vi "knrm-robotics-ultrasonic-scan.vi"() -> ()   [LabVIEW 2015]
uses:
  <userlib>/KNR OS 3.0 LabVIEW Toolkit/Type Definition/Ultrasonic Port Number.ctl
  <userlib>/KNR OS 3.0 LabVIEW Toolkit/Type Definition/Resource.ctl
  <userlib>/KNR OS 3.0 LabVIEW Toolkit/Type Definition/RC Servo Port.ctl
  <vilib>/ptbypt/NI_PtbyPt.lvlib
panel:
  out "output array":u16[](array[numeric])
  in  "?":bool
  in  "?":bool
  out "x-y":u32
  in  "Port Number":T1 items=["US1-US4"=0, "US5-US8"=2]
  in  "RC Pulse Width (uS)":u16[](array[numeric])=[1500, 1500, 1500, 1500, 1500, 1500, 1500]
  out "US":dbl(slide)=299.99420158565044 scale=0.0..300.0
  out "Ultrasonic output":T2
  out "XY Graph":cluster{dbl[], dbl[]}(graph)={[52.83510722219944, 52.41501941107636, 18.825090961382138, 18.810750829633513, 18.842068219739453, 18.867520707739345, 18.86999233966576, 19.343794430132927, 19.299396729094312, 19.249120244854563, 19.192980292117813, 19.56923700536949, 19.550257015140925, 20.0268746752987, 19.94313209159437, 19.853314636661487, 19.757449669766896, 20.476600911619304, 32.61215421079407, 32.42225574220841, 32.62586723383785, 32.42968403430184, 32.65326536183423, 33.19253900698759, 32.94158974146576, 33.80108407369108, 37.79584583915372, 37.468367050903275, 36.76560921195627, 36.403821071494754, 35.70408342661834, 35.309448959916324, 30.390512880027405, 33.7842674842371, 33.026100281524855, 32.632293705492096, 31.8534734091588, 31.444722619895053, 31.310542727675877, 30.878844889448313, 29.345981113135775, 28.61370061639986, 28.17523999703333, 27.351455120555766, 26.58100847356183, 26.092549408742254, 25.633197609818932, 25.16603769058929, 25.173776355470487, 24.6820024593776, 24.149598305560747, 23.64363348068164, 22.855607283966688, 22.072898695449073, 21.548232931052418, 20.99779051069682, 20.4712305073856, 19.938434768952572, 19.39956559014096, 18.837099698165826, 18.287094309926037, 17.731518495608384, 17.1463576277358, 16.58094778294143, 16.010487220829134, 15.253730460161847, 14.68050882655889, 14.08939689452119, 13.50152896715735, 12.916257579894289, 12.327051775449814, 11.734091031619695, 11.13755596999065, 10.537628300921224, 9.934490768191035, 9.328327093335284, 8.731784028189727, 8.119248646656601, 7.504240063332757, 6.8869456157904345, 6.2675533378981925, 5.6543103020243946, 5.030399780002455, 4.3631046269165985, 3.7422752021515957, 3.120305844107791, 2.496188223621293, 1.785636799859872, 1.1907267982129588, 0.5954540896484806, 2.066038963463892e-15, -0.5888612411470842, -1.163760162118542, -1.7451971139043094, -2.3249046746875894, -2.9018096075419657, -3.446123927161177, -4.017822965793698, -4.588298136629306, -5.157375667404677, -5.730845630561522, -6.375830717568115, -6.979443065564002, -7.555304639800326, -8.125294747449619, -8.692809811607347, -9.252943998005462, -9.814703824821812, -10.511433242759157, -97.66855855808836, -12.115630210935187, -14.780776897049115, -15.03243125118948, -16.11558635268566, -20.83347185044012, -21.98075621495253, -25.193747403909317, -26.09141148542781, -26.981127870254667, -27.86262554216021, -25.72212889790534, -26.495751500330893, -27.261303240179316, -28.018550922974622, -28.76726388373698, -29.260992311107042, -29.703255042663816, -30.153894378895316, -30.572810483455903, -31.251091419621243, -31.93089026416236, -32.61268695568148, -33.2624749197111, -33.90213081165937, -34.245188616933525, -34.85886894020428, -35.869539315624316, -36.46860682740769, -37.056565648272105, -37.633236680265036, -38.1984442638038, -38.75201623118319, -39.293783959019336, -39.823582419614134, -40.688540608559144, -41.198270803183775, -41.69545160542513, -42.698360226241675, -43.175788543019294, -43.64006509635344, -44.09104846310844, -44.874017063377195, -45.3012949795156, -45.760672049510696, -46.57732247552712, -46.966699693554176, -52.016338848904994, -52.90258478875593, -53.2864354783321, -57.421220074576965, -82.14554405908432, -82.65483424315623, -53.743915627302584, -54.04049206105783, -54.320607237429286, -54.252457958663086, -54.49789897377209, -55.06135718998163, -86.91802410081984, -87.22721920998029, -57.39292961361045, -57.56080538417302, -84.61127588015269, -87.43054222606335, -87.60457982125371, -65.41196662411174, -65.50188079298516, -67.25229239181644, -67.4580059883256, -67.33432889952226, -67.49912463128567], [0.0, 0.9149075670341228, 0.6573866621236092, 0.9858296776277172, 1.317565761028515, 1.6506941707678109, 1.9833161143297424, 2.375119305299923, 2.712353325559518, 3.048761136720991, 3.384240265706206, 3.8038743386930016, 4.155535410903584, 4.623568330184559, 4.972381294834969, 5.319679623974433, 5.665357527167541, 6.260325150666395, 10.596331239671903, 11.163877937181766, 11.874844540237977, 12.448589368330708, 13.192775565335738, 14.08939689452119, 14.666540692565961, 15.761704357503108, 18.434265728166686, 19.091086563433738, 19.548621178777296, 20.178967527396583, 20.613762177526947, 21.21605735957737, 18.990100087534795, 21.939759834879325, 22.276385917980576, 22.849378041658824, 23.142903096441774, 23.69529808458086, 24.462476991257596, 25.00519555498049, 24.62420192856765, 24.873510465680386, 25.36910004239107, 25.50564452773545, 25.668981505970372, 26.09254940874225, 26.543953164351468, 26.98727137468978, 27.958311065896748, 28.39339585621924, 28.780370540359066, 29.19745575545069, 29.25384329180434, 29.291725911947594, 29.65859822440211, 29.987952663840147, 30.349847327677153, 30.702497134012567, 31.0457946622992, 31.350198534648506, 31.674176467595604, 31.988506139556034, 32.24760857477566, 32.541942310033185, 32.8263634544222, 32.711730535404534, 32.972962684076684, 33.19253900698759, 33.41745684763044, 33.64800137815105, 33.86829640149636, 34.07827481366822, 34.277872653208185, 34.46702912068076, 34.64568659719358, 34.81379066194859, 35.02127289601618, 35.16832963030732, 35.30467375070981, 35.43026372548378, 35.545061298706294, 35.69991023384921, 35.79315428611765, 35.53463558310762, 35.60537016126978, 35.66525899876386, 35.69715469994275, 34.07197985276371, 34.09795418438132, 34.113541948840066, 33.74097682535648, 33.735837911157894, 33.32573076299372, 33.300344677436904, 33.247685831376614, 33.16783558686001, 32.787678997428294, 32.72254211969623, 32.64743763864413, 32.56238843182445, 32.50124063563915, 32.80080552321191, 32.835697993643045, 32.72561977016228, 32.5887772524299, 32.44200787745185, 32.26885054669531, 32.10244970506474, 32.350865043356556, 283.65009017131854, 33.28742042700667, 38.50524026218143, 37.20657296470336, 37.965942235611514, 46.79274390418685, 47.137883820999214, 51.65483708601368, 51.20727828475838, 50.744121250481506, 50.26550706530237, 44.55203413000772, 44.096335591458654, 43.62720488191764, 43.14478490314336, 42.649222604934685, 41.7890278444039, 40.8830232198667, 40.01556938720181, 39.13141295092422, 38.59188393270723, 38.05375318704697, 37.51660474840471, 36.94172092002333, 36.35558428558721, 35.46193091431041, 34.85886894020429, 34.638811474599436, 34.0075260369806, 33.365881577492594, 32.714073547253555, 32.05230049330367, 31.3807639981259, 30.699668618242033, 30.009221821902685, 29.561955154591352, 28.84733977759426, 28.123937221450483, 27.728639348003938, 26.979227005050628, 26.22159652819797, 25.45597869902849, 24.87407383327599, 24.087125807087233, 23.316226995194086, 22.717278059455737, 21.900931745370343, 23.159166160261293, 22.455814955220205, 21.52911741451913, 22.041941234483758, 29.89853291510958, 28.460341801798872, 17.46245673999011, 16.521836464188556, 15.576183476949357, 14.536902297427226, 13.587852310280022, 12.71191593536959, 18.474996350022376, 16.95525383525952, 10.119921992781398, 9.116735945401807, 11.891339337430969, 10.735120736730053, 9.207612367883806, 5.722805538545885, 4.580337700157324, 3.5245432959488956, 2.3556854774912677, 1.175325082839114, 8.266258692495226e-15]}
  in  "RC Power":bool
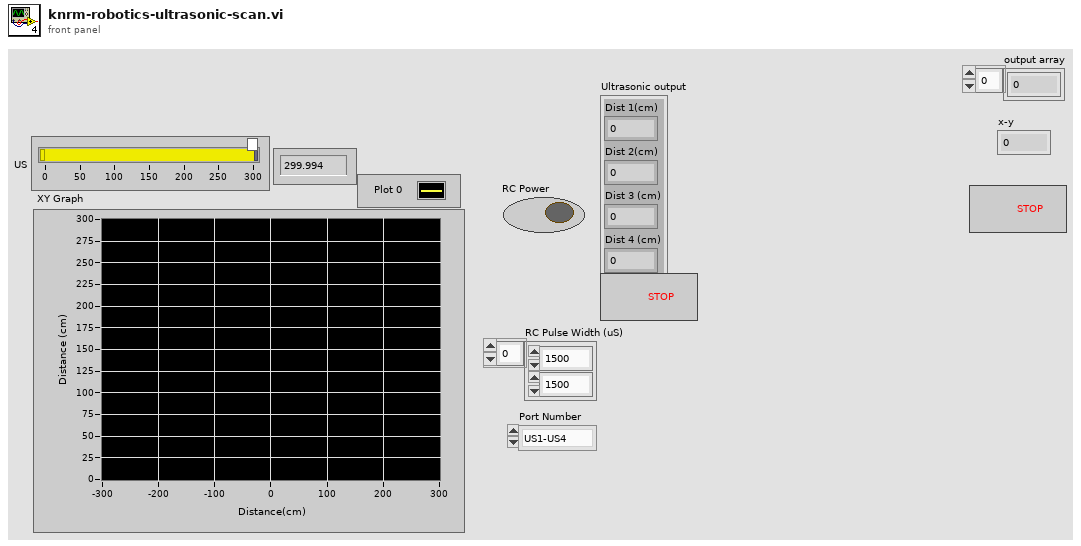
[diagram p1: front panel]
types:
  T1 = typedef "Ultrasonic Port Number.ctl" = u16
  T2 = cluster{"Dist 1(cm)":dbl, "Dist 2(cm)":dbl, "Dist 3 (cm)":dbl, "Dist 4 (cm)":dbl}
  T3 = typedef "Resource.ctl" = enum16{"KNRm_DDRC", "KNRm_DDDD", "KNRm_DDDR", "KNRm_DDDC", "KNR"}
  T4 = typedef "KNR3 Reference.ctl" = cluster{"FPGA Session":refnum<class "FPGA Interface Base.lvclass">, "Resource":T3}
  T5 = typedef "RC Servo Port.ctl" = u16
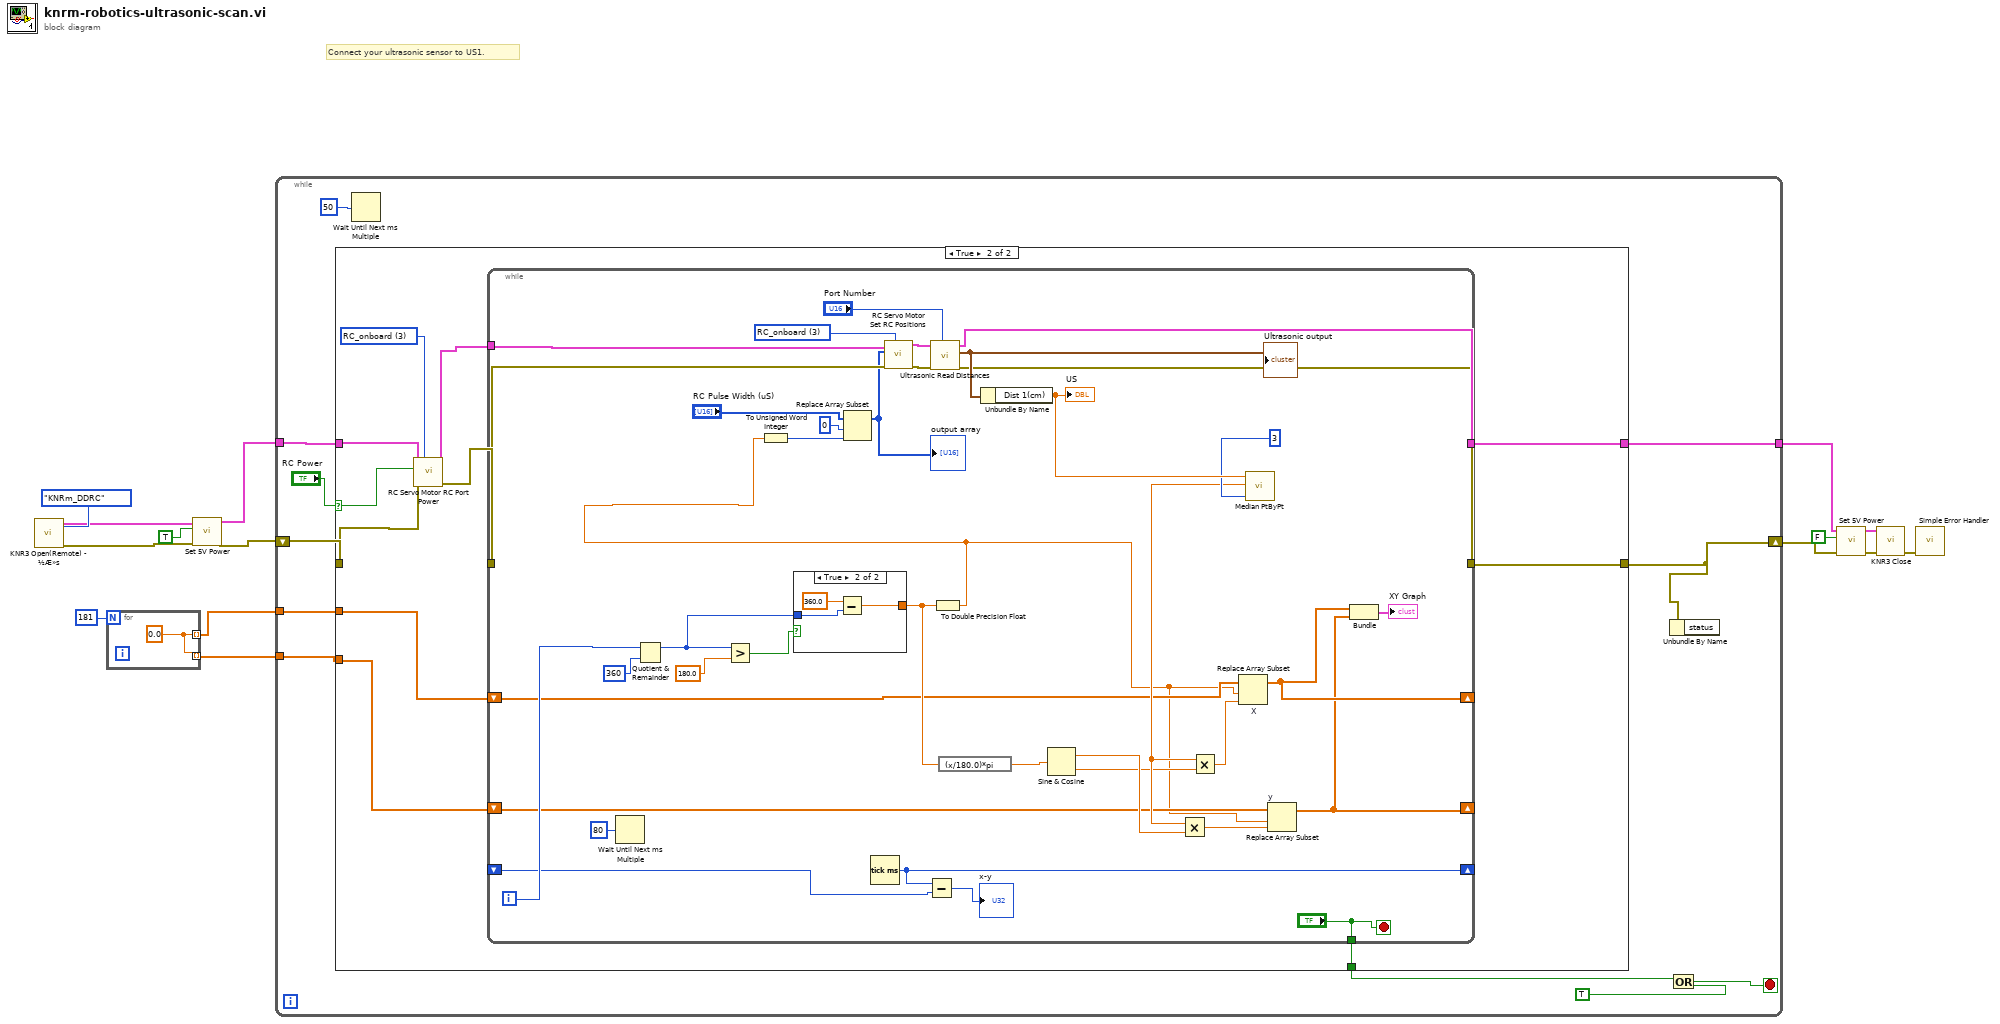
[diagram p0: block diagram]
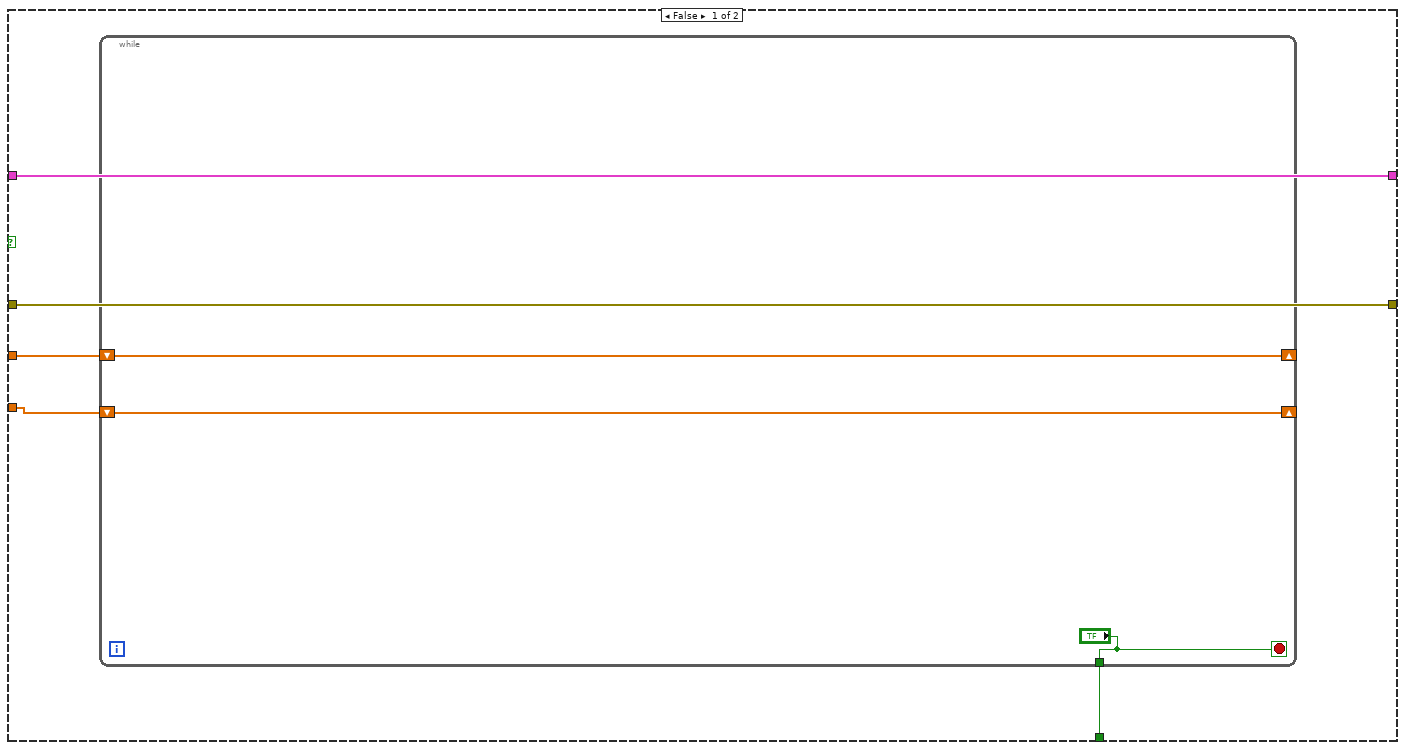
[diagram p2: hidden frame]
diagram:
  # "Connect your ultrasonic sensor to US1."
  n1 = call "KNR3 Open(Remote) - ½Æ»s.vi"("Resource"=Resource."KNRm_DDRC") -> ("error out"=w4:errorcluster, "KNR out"=w5:T4)  [unwired: 9 in]
  n2 = for {
    N: 181 -> [_]
    tunnel: [w16] -> w2 mode=indexing
    tunnel: [w16] -> w1 mode=indexing
    w16 = 0.0
  }
  n3 = call <userlib>:"Set 5V Power.vi"("error in (no error)"=w4, "5V Power(T)"=TRUE ("5V Power"), "KNR in"=w5) -> ("error out"=w13:errorcluster, "KNR out"=w14:T4)  [unwired: 7 in]
  n4 = while {
    tunnel: w14 -> [w27]
    shift-right: [w23] -> w12
    shift-left: w13 -> [w26]
    tunnel: [w22] -> w7
    tunnel: w2 -> [w21]
    tunnel: w1 -> [w20]
    stop <- w17 stop-if-true
    n5 = case shown="True" "RC Power" {
      selector: "RC Power" -> [_ w43]
      tunnel: [w31 w42] -> w22
      tunnel: w27 -> [w31 w40]
      tunnel: w26 -> [w32 w44]
      tunnel: [w32 w41] -> w23
      tunnel: w21 -> [w30 w38]
      tunnel: w20 -> [w29 w37]
      tunnel: [w28 w36] -> w18
      frame False {
        n6 = while {
          shift-right: [w35] -> _
          shift-left: w30 -> [w35]
          shift-right: [w34] -> _
          shift-left: w29 -> [w34]
          tunnel: ["?"] -> w28
          stop <- "?" stop-if-true
        }
      }
      frame True {
        w39 = T5 3 items=["RC_onboard"=3, "RC_box"=9] ("Port (RC_onboard)")
        n7 = call <userlib>:"RC Servo Motor RC Port Power.vi"("Port (RC_onboard)"=w39, "error in (no error)"=w44, "RC Power(F)"=w43, "KNR in"=w40) -> ("error out"=w45:errorcluster, "KNR out"=w46:T4)  [unwired: 6 in]
        n8 = while {
          tunnel: w46 -> [w71]
          tunnel: w45 -> [w82]
          tunnel: [w74] -> w42
          tunnel: [w73] -> w41
          shift-right: [w49] -> _
          shift-left: w38 -> [w59]
          shift-right: [w48] -> _
          shift-left: w37 -> [w58]
          shift-right: [w53] -> _
          shift-left: _ -> [w52]
          tunnel: ["?"] -> w36
          i -> [w65]
          stop <- "?" stop-if-true
          w70 = T5 3 items=["RC_onboard"=3, "RC_box"=9] ("Port (RC_onboard)")
          n9 = Wait Until Next ms Multiple(millisecond multiple=u32 80) -> ()  [unwired: 1 out]
          n10 = Quotient & Remainder(x=w65, y=360) -> (x-y*floor(x/y)=w61:i32)  [unwired: 1 out]
          n11 = Greater?(x=w61, y=180.0) -> (0:w62:bool)
          n12 = case shown="True" w62 {
            tunnel: w61 -> [w85 w87]
            tunnel: [w85 w86] -> w60
            frame False {
            }
            frame True {
              n13 = Subtract(x=360.0, y=w87) -> (x-y=w86:dbl)
            }
          }
          n14 = Tick Count (ms)() -> (millisecond timer value=w53:u32)
          n15 = Subtract(x=w53, y=w52) -> (x-y=→"x-y":u32)
          n16 = To Double Precision Float(number=w60) -> (double precision float=w47:dbl)
          n17 = To Unsigned Word Integer(number=w47) -> (unsigned 16bit integer=w78:u16)
          n18 = Replace Array Subset(array="RC Pulse Width (uS)", new element=w78, index=0) -> (w77:u16[])
          "output array" <- w77
          n19 = call <userlib>:"RC Servo Motor Set RC Positions.vi"("Port (RC_onboard)"=w70, "error in (no error)"=w82, "RC Pulse Width (1500 uS)"=w77, "KNR in"=w71) -> ("error out"=w83:errorcluster, "KNR out"=w72:T4)  [unwired: 6 in]
          n20 = call <userlib>:"Ultrasonic Read Distances.vi"("Port (US1-US4 for KNR)"="Port Number", "error in (no error)"=w83, "KNR in"=w72) -> ("error out"=w73:errorcluster, "Ultrasonic output"=w81:T2, "KNR out"=w74:T4)  [unwired: 6 in]
          "Ultrasonic output" <- w81
          n21 = expression code="(x/180.0)*pi"(w60) -> (w76:dbl)
          n22 = Unbundle By Name(w81) -> ("Dist 1(cm)"=w69:dbl)
          "US" <- w69
          n23 = Sine & Cosine(0:w76) -> (1:w75:dbl, 2:w57:dbl)
          n24 = call <vilib>:"Median PtByPt.vi"("sample length"=3, "x"=w69) -> ("median"=w67:dbl)  [unwired: 2 in, 1 out]
          n25 = Multiply(x=w67, y=w75) -> (x*y=w54:dbl)
          n26 = Multiply(x=w67, y=w57) -> (x*y=w55:dbl)
          n27 = Replace Array Subset "X"(array=w59, new element=w55, index=w47) -> (w49:dbl[])
          n28 = Replace Array Subset "y"(array=w58, new element=w54, index=w47) -> (w48:dbl[])
          n29 = Bundle(w49, w48) -> (→"XY Graph":cluster{dbl[], dbl[]})  [unwired: 1 in]
        }
      }
    }
    n30 = Wait Until Next ms Multiple(millisecond multiple=u32 50) -> ()  [unwired: 1 out]
    n31 = Unbundle By Name(w23) -> ()  [unwired: 1 out]
    n32 = Or(x=w18, y=TRUE) -> (x .or. y?=w17:bool)
  }
  n33 = call <userlib>:"Set 5V Power.vi"("error in (no error)"=w12, "5V Power(T)"=FALSE ("5V Power"), "KNR in"=w7) -> ("error out"=w11:errorcluster, "KNR out"=w8:T4)  [unwired: 7 in]
  n34 = call <userlib>:"KNR3 Close.vi"("error in (no error)"=w11, "KNR in"=w8) -> ("error out"=w9:errorcluster)  [unwired: 9 in]
  n35 = call <vilib>:"Simple Error Handler.vi"("error in (no error)"=w9) -> ()  [unwired: 4 in, 5 out]
